vi "FGV Map Delete Data.vi"(8 "error in (no error)":errorcluster, 11 "Instance Key":string) -> (0 "error out":errorcluster, 2 "Data Deleted ?":bool, 3 "Deleted Data":variant)   [LabVIEW 2020, in "FGV Map.lvlib"]
uses:
  FGV Map.lvlib
  Controls/FGV Map Core State.ctl
panel:
  in  "Data Key":string
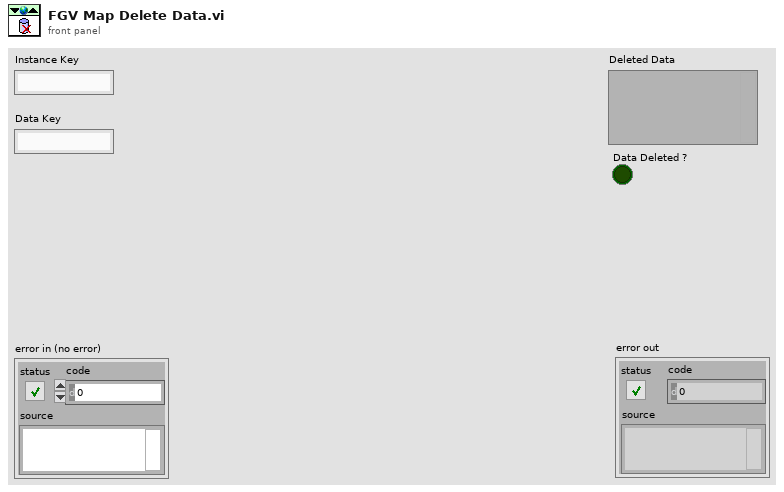
[diagram p1: front panel]
types:
  T1 = typedef "FGV Map.lvlib/FGV Map Core State.ctl" = enum16{"Init", "Set Instance (Unlock)", "Get Instance", "Get Instance (Lock)", "Unlock", "Delete Instance"}
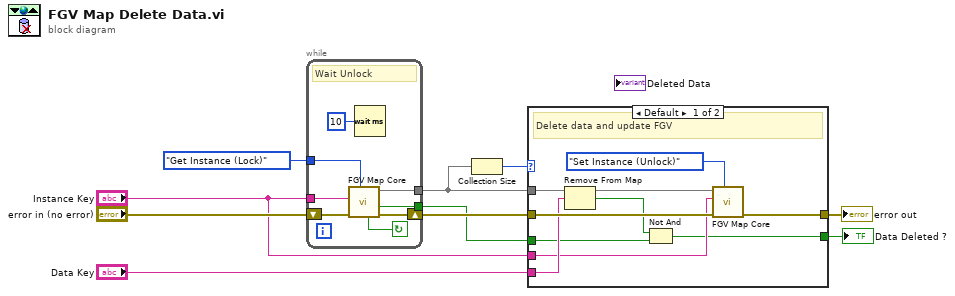
[diagram p0: block diagram]
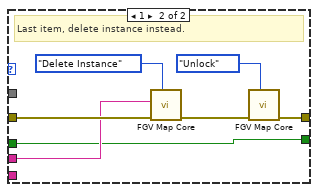
[diagram p2: hidden frame]
diagram:
  n1 = while {
    tunnel: FGV_Map_Core_State."Get Instance (Lock)" ("FGV State") -> [w17]
    tunnel: [w16] -> w7
    tunnel: "Instance Key" -> [w14]
    shift-right: [w15] -> w3
    shift-left: "error in (no error)" -> [w18]
    tunnel: [w11] -> w2
    stop <- w13 continue-if-true
    # "Wait Unlock"
    n2 = call "FGV Map Core.vi"("FGV State"=w17, "error in"=w18, "Instance Key"=w14) -> ("error out"=w15:errorcluster, "Instance Not Found ?"=w11:bool, "Instance Out"=w16:map{string, variant}, "Was Locked ?"=w13:bool)  [unwired: 4 in, 1 out]
    n3 = Wait (ms)(milliseconds to wait=u32 10) -> ()  [unwired: 1 out]
  }
  n4 = Collection Size(1:w7) -> (0:w8:i32)
  n5 = case shown="Default" w8 {
    tunnel: w7 -> [w28 _]
    tunnel: w3 -> [w27 w35]
    tunnel: "Data Key" -> [w26 _]
    tunnel: "Instance Key" -> [w23 w30]
    tunnel: [w22 w32] -> w4
    tunnel: w2 -> [w21 w29]
    tunnel: [w19 w29] -> w1
    frame Default {
      # "Delete data and update FGV"
      n6 = Remove From Map(10:w26, 11:w28) -> (2:w20:bool, 3:w25:map{string, variant})  [unwired: 1 out]
      n7 = Not And(1:w21, 2:w20) -> (0:w19:bool)
      n8 = call "FGV Map Core.vi"("FGV State"=FGV_Map_Core_State."Set Instance (Unlock)", "error in"=w27, "Instance Key"=w23, "Instance In"=w25) -> ("error out"=w22:errorcluster)  [unwired: 3 in, 4 out]
    }
    frame 1 {
      # "Last item, delete instance instead."
      n9 = call "FGV Map Core.vi"("FGV State"=FGV_Map_Core_State."Delete Instance", "error in"=w35, "Instance Key"=w30) -> ("error out"=w33:errorcluster)  [unwired: 4 in, 4 out]
      n10 = call "FGV Map Core.vi"("FGV State"=FGV_Map_Core_State."Unlock", "error in"=w33) -> ("error out"=w32:errorcluster)  [unwired: 5 in, 4 out]
    }
  }
  "error out" <- w4
  "Data Deleted ?" <- w1
